vi "Set Stop Trigger (In Range).vi"(7 "Post-Trigger Duration (0 s)":dbl, 8 "error in (no error)":errorcluster, 9 "Trigger Channel":string, 10 "Range Options":T1, 11 "Data Logging Specification Ref in":T2) -> (0 "error out":errorcluster, 3 "Data Logging Specification Ref out":T2)   [LabVIEW 2020, in "NI_VS Data Logging API.lvlib"]
doc: "Specifies a trigger condition on which to stop logging data. You also can specify whether to continue logging channel data for a set period of time after the trigger condition occurs.\n\nYou must manually select the polymorphic instance to use."
uses:
  <vilib>/NI VeriStand/Execution/DataLogging/NI_VS Data Logging API.lvlib
  <vilib>/NI VeriStand/Execution/DataLogging/DataLoggingSpecification Ref.ctl
  NationalInstruments.VeriStand.ClientAPI
  <vilib>/NI VeriStand/Execution/DataLogging/Range Options.ctl
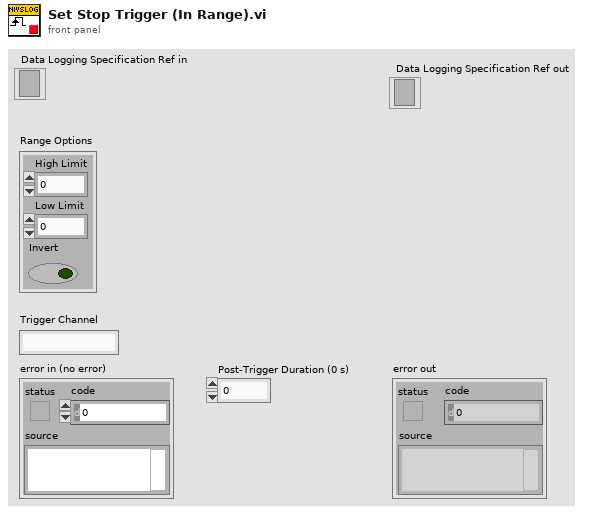
[diagram p1: front panel]
types:
  T1 = typedef "NI_VS Data Logging API.lvlib/Range Options.ctl" = cluster{"High Limit":dbl, "Low Limit":dbl, "Invert":bool}
  T2 = typedef "NI_VS Data Logging API.lvlib/DataLoggingSpecification Ref.ctl" = refnum<k24>
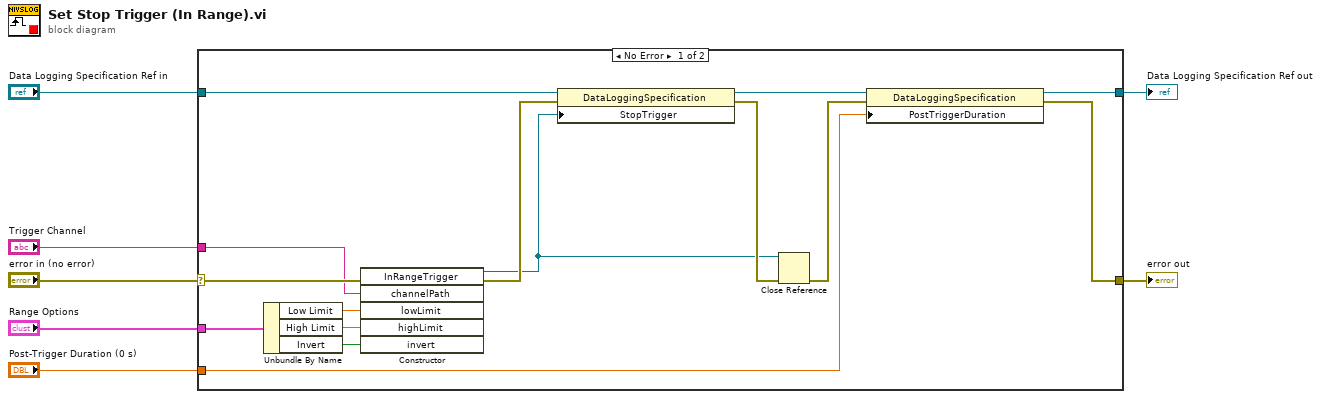
[diagram p0: block diagram]
diagram:
  n1 = case shown="No Error" "error in (no error)" {
    selector: "error in (no error)" -> [w12 w24]
    tunnel: "Data Logging Specification Ref in" -> [w21 w23]
    tunnel: "Post-Trigger Duration (0 s)" -> [w20 _]
    tunnel: [w17 w23] -> w5
    tunnel: [w16 w24] -> w4
    tunnel: "Range Options" -> [w8 _]
    tunnel: "Trigger Channel" -> [w9 _]
    frame No Error {
      n2 = Unbundle By Name(w8) -> ("Low Limit"=w15:dbl, "High Limit"=w14:dbl, "Invert"=w13:bool)
      n3 = constructor class="InRangeTrigger"(error in=w12, "channelPath"=w9, "lowLimit"=w15, "highLimit"=w14, "invert"=w13) -> (reference out=w10:refnum<k24>, error out=w11:errorcluster)  [unwired: 2 in, 5 out]
      n4 = property class="DataLoggingSpecification"(reference=w21, error in=w11, "StopTrigger"=w10) -> (reference out=w19:T2, error out=w22:errorcluster)
      n5 = Close Reference(reference=w10, error in (no error)=w22) -> (error out=w18:errorcluster)
      n6 = property class="DataLoggingSpecification"(reference=w19, error in=w18, "PostTriggerDuration"=w20) -> (reference out=w17:T2, error out=w16:errorcluster)
    }
    frame Error {
    }
  }
  "error out" <- w4
  "Data Logging Specification Ref out" <- w5
